vi "programa12.vi"() -> ()   [LabVIEW 2011]
uses:
  <vilib>/express/express arith-compare/Formula/XNode/ExpressFormulaBlockNode.xnode
panel:
  out "Menor":dbl
  out "Mayor":dbl
  out "Promedio":dbl
  out "Contador":dbl
  out "Numero Par":dbl
  # "Elabore un programa donde se generen y presenten 5 numeros pares"
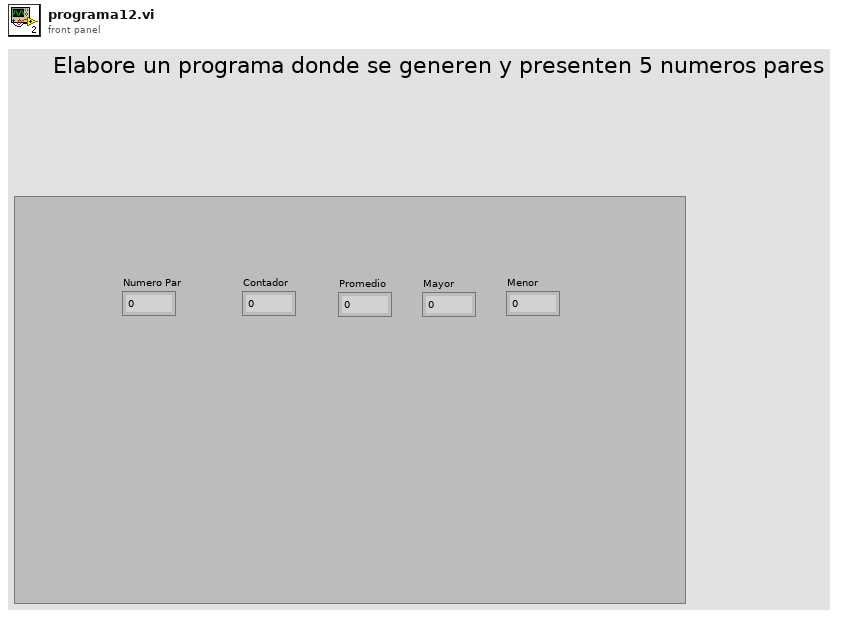
[diagram p1: front panel]
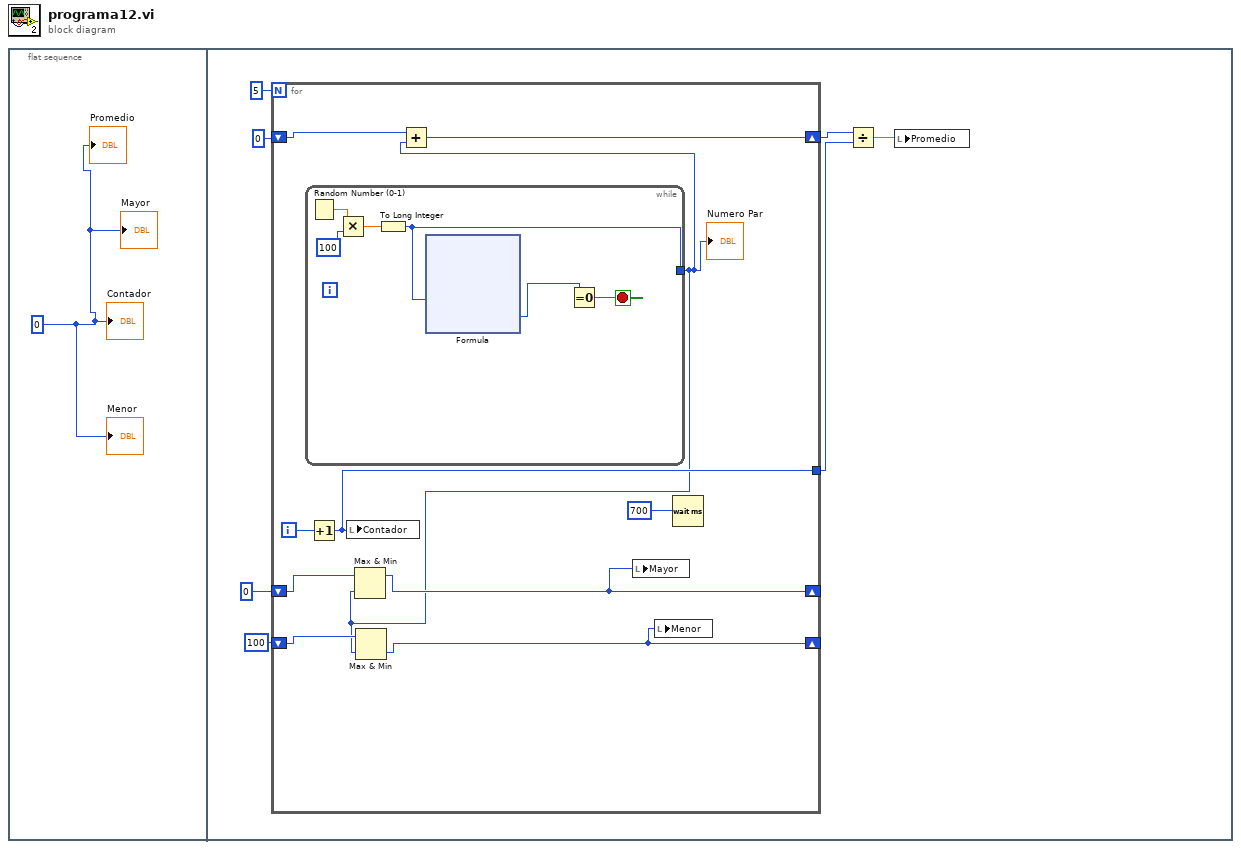
[diagram p0: block diagram]
diagram:
  n1 = flat-sequence {
    frame #0 {
      w1 = 0
      "Contador" <- w1
      "Promedio" <- w1
      "Mayor" <- w1
      "Menor" <- w1
    }
    frame #1 {
      n2 = for {
        N: 5 -> [_]
        shift-right: [w15] -> w6
        shift-left: 0 -> [w16]
        tunnel: [w14] -> w4
        shift-right: [w11] -> _
        shift-left: 0 -> [w13]
        shift-right: [w10] -> _
        shift-left: 100 -> [w12]
        i -> [w18]
        n3 = while {
          tunnel: [w19] -> w9
          stop <- w20 stop-if-true
          n4 = Random Number (0-1)() -> (number: 0 to 1=w22:dbl)
          n5 = Multiply(x=w22, y=100) -> (x*y=w23:dbl)
          n6 = To Long Integer(number=w23) -> (32bit integer=w19:i32)
          n7 = xnode "Formula"("X1"=w19) -> ("Result"=w21:i32)  [unwired: 1 in, 1 out]
          n8 = Equal To 0?(x=w21) -> (x = 0?=w20:bool)
        }
        "Numero Par" <- w9
        n9 = Increment(x=w18) -> (x+1=w14:i32)
        n10 = local write "Contador"(w14) -> ()
        n11 = Max & Min(x=w13, y=w9) -> (max(x,y)=w11:i32)  [unwired: 1 out]
        n12 = Max & Min(x=w12, y=w9) -> (min(x,y)=w10:i32)  [unwired: 1 out]
        n13 = Add(x=w16, y=w9) -> (x+y=w15:i32)
        n14 = local write "Mayor"(w11) -> ()
        n15 = local write "Menor"(w10) -> ()
        n16 = Wait (ms)(milliseconds to wait=700) -> ()  [unwired: 1 out]
      }
      n17 = Divide(x=w6, y=w4) -> (x/y=w5:dbl)
      n18 = local write "Promedio"(w5) -> ()
    }
  }
